vi "ReadLine.vi"(8 "error in (no error)":errorcluster, 9 "Timeout":i32=2000, 10 "NumOfBytes":i32=100, 11 "ClientBase in":refnum<class "TCP.lvclass">) -> (0 "error out":errorcluster, 1 "Length":i32, 2 "Data":string, 3 "ClientBase out":refnum<class "TCP.lvclass">)   [LabVIEW 2020, in "TCP.lvlib" / "TCP.lvclass"]
uses:
  TCP.lvclass
  TCP.lvclass/TCP.ctl
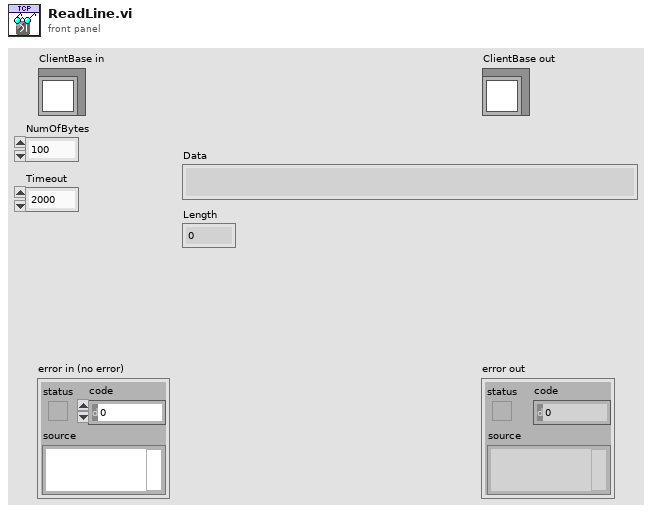
[diagram p1: front panel]
types:
  T1 = enum16{"Standard", "Buffered", "CRLF", "Immediate"}
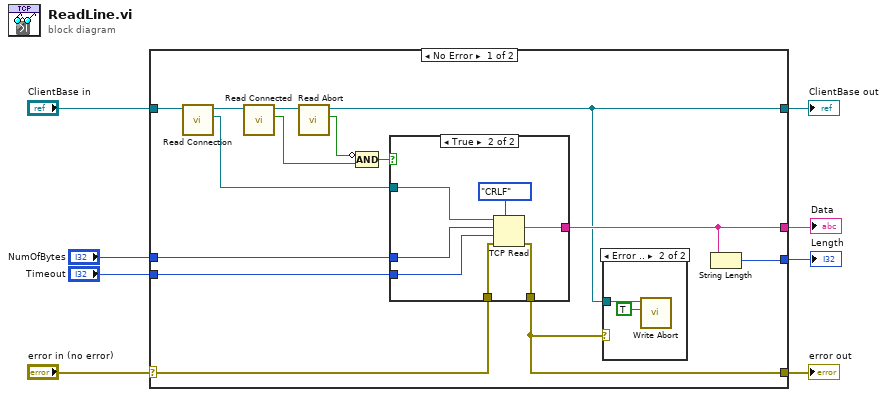
[diagram p0: block diagram]
diagram:
  n1 = case shown="No Error" "error in (no error)" {
    selector: "error in (no error)" -> [w22 w34]
    tunnel: [w10 w34] -> w7
    tunnel: [w9 w33] -> w5
    tunnel: "ClientBase in" -> [w12 w33]
    tunnel: [w21 _] -> w4
    tunnel: [w20 _] -> w3
    tunnel: "Timeout" -> [w18 _]
    tunnel: "NumOfBytes" -> [w17 _]
    frame No Error {
      n2 = call "Read Connection.vi"("ClientBase in"=w12) -> ("Connection ID"=w14:refnum<k5>, "ClientBase out"=w16:refnum<class "TCP.lvclass">)  [unwired: 8 in, 1 out]
      n3 = call "Read Connected.vi"("ClientBase in"=w16) -> ("Connected"=w15:bool, "ClientBase out"=w13:refnum<class "TCP.lvclass">)  [unwired: 8 in, 1 out]
      n4 = call "Read Abort.vi"("ClientBase in"=w13) -> ("Abort"=w11:bool, "ClientBase out"=w9:refnum<class "TCP.lvclass">)  [unwired: 8 in, 1 out]
      n5 = Compound Arithmetic op=AND(invert w11, w15) -> (w19:bool)
      n6 = case shown="True" w19 {
        tunnel: w14 -> [_ w32]
        tunnel: w22 -> [w25 w31]
        tunnel: [w25 w30] -> w10
        tunnel: [_ w28] -> w21
        tunnel: w18 -> [_ w27]
        tunnel: w17 -> [_ w26]
        frame False {
        }
        frame True {
          n7 = TCP Read(connection ID=w32, bytes to read=w26, error in (no error)=w31, 7:T1."CRLF" ("mode (standard)"), 9:w27) -> (data out=w28:string, error out=w30:errorcluster)  [unwired: 1 out]
        }
      }
      n8 = case shown="Error .." w10 {
        tunnel: w9 -> [_ w24]
        frame No Error {
        }
        frame Error {
          n9 = call "Write Abort.vi"("Abort"=TRUE, "ClientBase in"=w24) -> ()  [unwired: 8 in, 2 out]
        }
      }
      n10 = String Length(string=w21) -> (length=w20:i32)
    }
    frame Error {
    }
  }
  "error out" <- w7
  "ClientBase out" <- w5
  "Data" <- w4
  "Length" <- w3
